vi "dfd_Kaiser Beta from Order.vi"(9 "delta f [Hz]":dbl=0.1 format="%.2f", 11 "order":i32) -> (1 "r [dB]":dbl, 3 "beta":dbl format="%.2f")   [LabVIEW 2017, in "NI_DigFilter_Process.lvlib"]
uses:
  <vilib>/addons/Digital Filter Design/NI_DigFilter_Process.lvlib
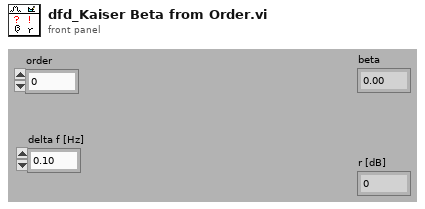
[diagram p1: front panel]
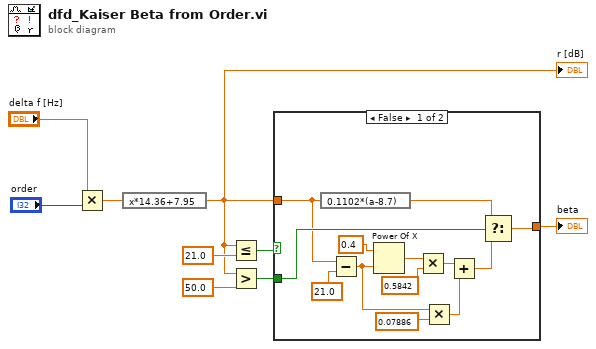
[diagram p0: block diagram]
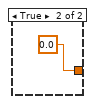
[diagram p2: hidden frame]
diagram:
  n1 = Multiply(x="delta f [Hz]", y="order") -> (x*y=w2:dbl)
  n2 = expression code="x*14.36+7.95"(w2) -> (w5:dbl)
  "r [dB]" <- w5
  n3 = Less Or Equal?(x=w5, y=21.0) -> (x <= y?=w4:bool)
  n4 = Greater?(x=w5, y=50.0) -> (0:w3:bool)
  n5 = case shown="False" w4 {
    tunnel: [w10 0.0] -> w8
    tunnel: w5 -> [w11 _]
    tunnel: w3 -> [w12 _]
    frame False {
      n6 = expression code="0.1102*(a-8.7)"(w11) -> (w22:dbl)
      n7 = Subtract(x=w11, y=21.0) -> (x-y=w16:dbl)
      n8 = Power Of X(1:w16, 2:0.4 ("y")) -> (0:w19:dbl)
      n9 = Multiply(x=w19, y=0.5842) -> (x*y=w15:dbl)
      n10 = Multiply(x=w16, y=0.07886) -> (x*y=w14:dbl)
      n11 = Add(x=w15, y=w14) -> (x+y=w13:dbl)
      n12 = Select(t=w22, s=w12, f=w13) -> (s? t:f=w10:dbl)
    }
    frame True {
    }
  }
  "beta" <- w8
